vi "PH_Tektronix_7000.Init.vi"(0 "i ref in":refnum<vi>, 5 "error in (no error)":errorcluster) -> (14 "i ref out":refnum<vi>, 19 "error out":errorcluster)   [LabVIEW 2014, in "PH_Tektronix_7000.lvlib"]
doc: "Initializes the connection to the hardware and queries the errors which are written to own attributes. The \"connection established\" flag is set to true in case of no error."
uses:
  PH_Tektronix_7000.lvlib
  PH_Basics/PH_Common/PH_Common.lvlib
  instr.lib/Tektronix7000Series/Tektronix 7000 Series - Driver np.lvlib
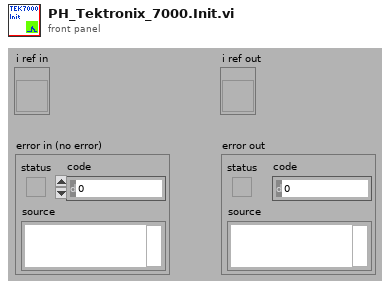
[diagram p1: front panel]
types:
  T1 = typedef "PH_Tektronix_7000.lvlib/PH_Tektronix_7000.i attribute.ctl" = cluster{"VISA Resource Name":refnum<visa-resource-name>, "IDN":cluster{"Instrument Driver":string, "Instrument Firmware":string, "Model":string, "Serial Number":string}, "Selftest":cluster{"Result":i32, "Message":string}, "Trigger Configuration":T2, "Acquisition Configuration":T3, "GUI Refs":T4, "State":T5, "Error Message":string, "Allow Prdc Loop?":bool, "Channel 1":T6, "Channel 2":T6, "Channel 3":T6, "Channel 4":T6, "Data CH 1":waveform(dbl), "Data CH 2":waveform(dbl), "Data CH 3":waveform(dbl), "Data CH 4":waveform(dbl), "Allow config?":bool, "Name Channel 1":string, "Name Channel 2":string, "Name Channel 3":string, "Name Channel 4":string, "Fetch Data before sending to PSDB?":bool, "Constructor passed?":bool, "Data taken at":timestamp, "Plot Colors":u32[], "Default VISA Resource":string}
  T2 = typedef "PH_Tektronix_7000.lvlib/PH_Tektronix_7000.Trigger Config.ctl" = cluster{"Source":u16, "Level [V]":dbl, "Slope":u16, "Coupling":u16, "Trigger Mode":u16}
  T3 = typedef "PH_Tektronix_7000.lvlib/PH_Tektronix_7000.Acquisition Config.ctl" = cluster{"Record Length":u32, "Timebase [s/div]":dbl, "Position [%]":dbl, "Acquisition Type":u16, "Average Waveforms":i32, "Envelope Waveforms":i32, "WfmDB Samples":i32, "Continuous?":bool, "Delay [s]":dbl, "Run?":bool}
  T4 = typedef "PH_Tektronix_7000.lvlib/PH_Tektronix_7000.GUI Refs.ctl" = cluster{"Graph":refnum<vi>, "State":refnum<vi>, "Delete":refnum<vi>, "VISA Resource":refnum<vi>, "Allow Configure":refnum<vi>, "Fetch Data":refnum<vi>, "Fetch before sending Data to PSDB":refnum<vi>, "Name Channel 1":refnum<vi>, "Name Channel 2":refnum<vi>, "Name Channel 3":refnum<vi>, "Name Channel 4":refnum<vi>, "Prdc Intervall [ms]":refnum<vi>, "Data taken":refnum<vi>, "Model":refnum<vi>, "Serial Number":refnum<vi>, "Firmware":refnum<vi>, "Driver":refnum<vi>, "Acquisition":refnum<vi>, "Trigger":refnum<vi>, "Cursor: D Time [s]":refnum<vi>, "Cursor: D Signal [V]":refnum<vi>, "Channel 1":refnum<vi>, "Channel 2":refnum<vi>, "Channel 3":refnum<vi>, "Channel 4":refnum<vi>}
  T5 = typedef "PH_StatusHandler.lvlib/PH_StatusHandler.Status.ctl" = i16
  T6 = typedef "PH_Tektronix_7000.lvlib/PH_Tektronix_7000.Channel Config.ctl" = cluster{"Enable Channel":bool, "Bandwidth":u16, "Input Impedance":u16, "Vertical Coupling":u16, "Probe Attenuation":dbl, "Range [V/div]":dbl, "Position [div]":dbl, "Bandwidth raw":string}
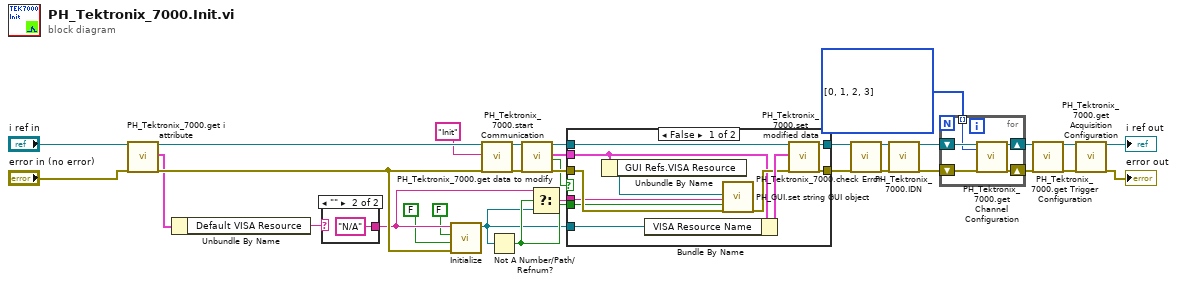
[diagram p0: block diagram]
diagram:
  w24 = u16[] [0, 1, 2, 3] items=["Channel 1", "Channel 2", "Channel 3", "Channel 4", "Math 1", "Math 2", "Math 3", "Math 4", "Reference 1", "Reference 2", "Reference 3", "Reference 4"]
  n1 = call "PH_Tektronix_7000.get i attribute.vi"("i ref in"="i ref in", "error in (no error)"="error in (no error)") -> ("i ref out"=w32:refnum<vi>, "i attribute"=w6:T1, "error out"=w31:errorcluster)  [unwired: 15 in]
  n2 = Unbundle By Name(w6) -> ("Default VISA Resource"=w1:string)
  n3 = case shown="\"\"" w1 {
    selector: w1 -> [w33 _]
    tunnel: [w33 "N/A"] -> w21
    frame Default {
    }
    frame "" {
    }
  }
  n4 = call "Initialize.vi"("error in (no error)"=w31, "Reset? ( Yes)"=FALSE, "ID Query? ( Yes)"=FALSE, "VISA resource name"=w21) -> ("VISA resource name out"=w7:refnum<visa-resource-name>)  [unwired: 4 in, 3 out]
  n5 = call "PH_Tektronix_7000.start Communication.vi"("i ref in"=w32, "Action"="Init", "error in"=w31) -> ("i ref out"=w14:refnum<vi>, "error out"=w13:errorcluster)  [unwired: 15 in]
  n6 = Not A Number/Path/Refnum?(number/path/refnum=w7) -> (NaN/Path/Refnum?=w8:bool)
  n7 = call "PH_Tektronix_7000.get data to modify.vi"("i ref in"=w14, "error in (no error)"=w13) -> ("i ref out"=w19:refnum<vi>, "i attribute"=w17:T1, "timed out"=w18:bool, "error out"=w20:errorcluster)  [unwired: 14 in]
  n8 = Select(t=w21, s=w8, f=w7) -> (s? t:f=w9:string)
  n9 = case shown="False" w18 {
    tunnel: [w45 w46] -> w15
    tunnel: w20 -> [w44 w46]
    tunnel: w19 -> [w43 w47]
    tunnel: [w42 w47] -> w16
    tunnel: w17 -> [w39 _]
    tunnel: w7 -> [w36 _]
    tunnel: w9 -> [w37 _]
    tunnel: w8 -> [w35 _]
    frame False {
      n10 = Unbundle By Name(w39) -> ("GUI Refs.VISA Resource"=w38:refnum<vi>)
      n11 = Bundle By Name(cluster=w39, "VISA Resource Name"=w36) -> (w41:T1)
      n12 = call "PH_GUI.set string GUI object.vi"("GUI object Ref"=w38, "Text"=w37, "Blinking? (false)"=w35, "error in"=w44) -> ("error out"=w40:errorcluster)  [unwired: 15 in]
      n13 = call "PH_Tektronix_7000.set modified data.vi"("i ref in"=w43, "i attribute"=w41, "error in (no error)"=w40) -> ("i ref out"=w42:refnum<vi>, "error out"=w45:errorcluster)  [unwired: 15 in]
    }
    frame True {
    }
  }
  n14 = call "PH_Tektronix_7000.check Error.vi"("i ref in"=w16, "error in"=w15) -> ("i ref out"=w5:refnum<vi>, "error out"=w3:errorcluster)  [unwired: 16 in]
  n15 = call "PH_Tektronix_7000.IDN.vi"("i ref in"=w5, "error IO"=w3) -> ("i ref out"=w4:refnum<vi>, "error out"=w2:errorcluster)  [unwired: 16 in]
  n16 = for {
    shift-right: [w49] -> w25
    shift-left: w2 -> [w52]
    shift-right: [w51] -> w26
    shift-left: w4 -> [w50]
    tunnel: w24 -> [w48] mode=indexing
    n17 = call "PH_Tektronix_7000.get Channel Configuration.vi"("i ref in"=w50, "Channel"=w48, "error IO"=w52) -> ("i ref out"=w51:refnum<vi>, "error out"=w49:errorcluster)  [unwired: 15 in]
  }
  n18 = call "PH_Tektronix_7000.get Trigger Configuration.vi"("i ref in"=w26, "error IO"=w25) -> ("i ref out"=w28:refnum<vi>, "error out"=w27:errorcluster)  [unwired: 16 in]
  n19 = call "PH_Tektronix_7000.get Acquisition Configuration.vi"("i ref in"=w28, "error IO"=w27) -> ("i ref out"=→"i ref out":refnum<vi>, "error out"=→"error out":errorcluster)  [unwired: 16 in]
